vi "(SubVI) Guess Center xc yc From Raw FEC_YCC.vi"(5 "Enum":enum16{"parity method", "max-min method"}(ring), 6 "avg range for QPD center (nm)":dbl=600.0, 7 "QPD array (V)":dbl[](array[numeric]), 8 "Stage array(um)":dbl[](array[numeric]), 9 "Read data?":bool) -> (0 "Best Fit for min":cluster{"X":dbl[], "Best Polynomial Fit":dbl[]}, 1 "Best Fit for max":cluster{"X":dbl[], "Best Polynomial Fit":dbl[]}, 2 "Guess-QPD-center (V)":dbl, 3 "Guess-stage-center(um)":dbl)   [LabVIEW 2014]
uses:
  <vilib>/Analysis/6fits.llb/Curve Fitting Criteria.ctl
  <vilib>/Analysis/6fits.llb/General Linear Fit Algorithm.ctl
  <vilib>/Utility/file.llb/Read From Spreadsheet File (DBL).vi
  <vilib>/Analysis/NI_AALPro.lvlib
panel:
  out "Guess-stage-center by avg (um)":dbl
  out "Guess-stage-center by fit (um)":dbl
  out "Xm for min QPD":dbl
  out "Xm for max QPD":dbl
  in  "file path (dialog if empty)":path
  in  "Tab Control":T1(tab)
  out "Raw":cluster{"all rows":dbl[], "all rows":dbl[]}(graph)
  out "Fit":cluster{"all rows":dbl[], "all rows":dbl[]}(graph)
  out "Raw+Fit":cluster{"all rows":dbl[], "all rows":dbl[]}[](graph)
  out "XY Graph":T2(graph)
  out "Polynomial Coefficients":dbl[](array[numeric])
  out "Best Fit for QPD":dbl[](array[numeric])
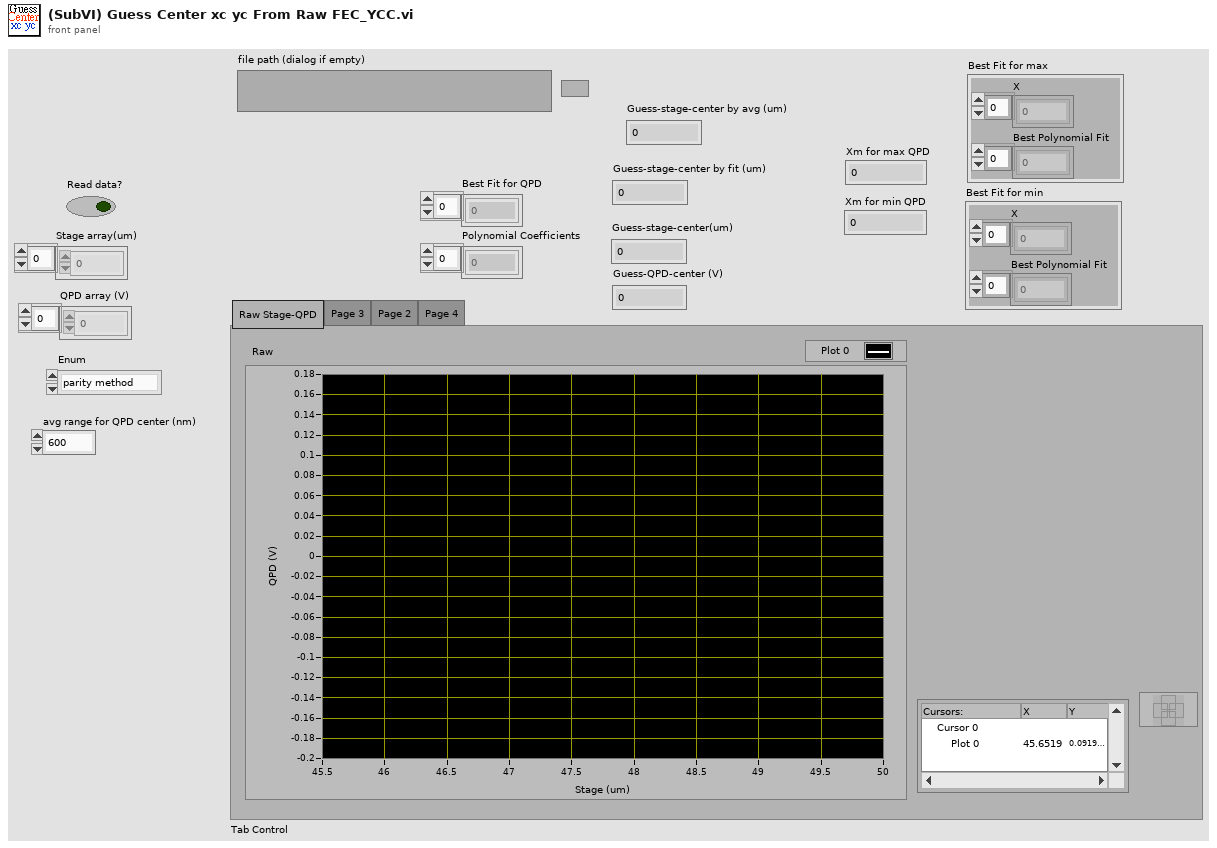
[diagram p1: front panel]
types:
  T1 = enum32{"Raw Stage-QPD", "Page 3", "Page 2", "Page 4"}
  T2 = cluster{"X":dbl[], "Best Polynomial Fit":dbl[]}[]
  T3 = typedef "NI_AALPro.lvlib/General Linear Fit Algorithm.ctl" = u16
  T4 = typedef "NI_AALPro.lvlib/Curve Fitting Criteria.ctl" = u16
  T5 = cluster{"all rows":dbl[], "Best Polynomial Fit":dbl[]}
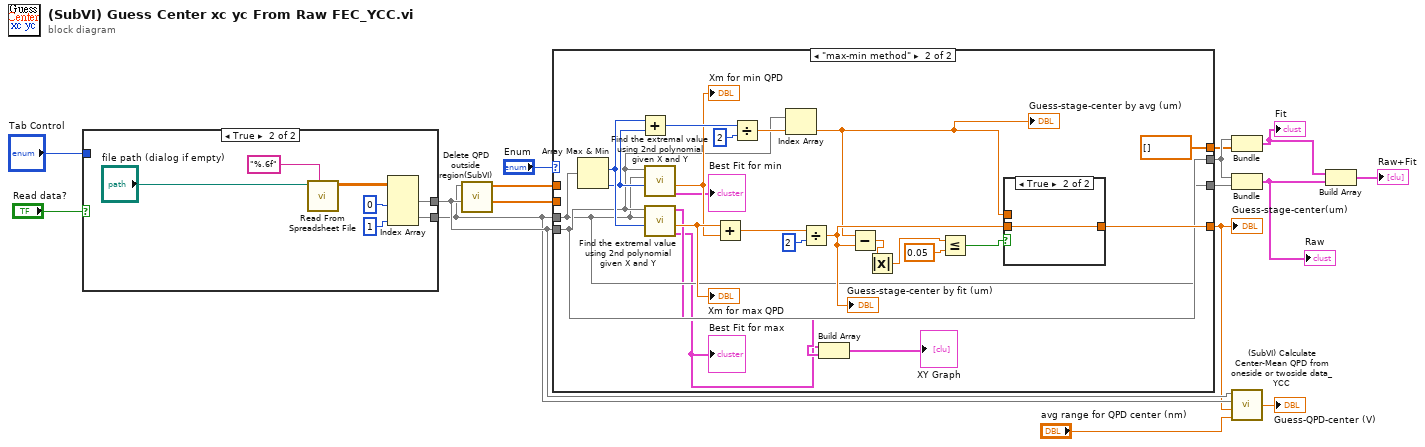
[diagram p0: block diagram]
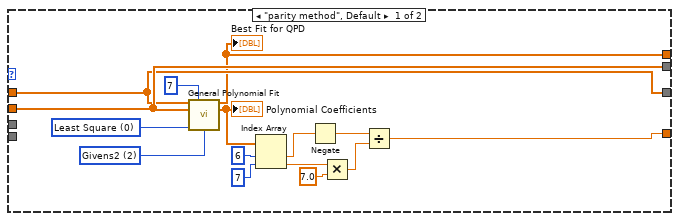
[diagram p2: hidden frame]
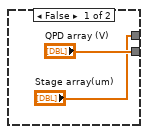
[diagram p4: hidden frame]
diagram:
  n1 = case shown="True" "Read data?" {
    tunnel: ["QPD array (V)" w20] -> w4
    tunnel: ["Stage array(um)" w21] -> w5
    tunnel: "Tab Control" -> [_ _]
    frame False {
    }
    frame True {
      n2 = call-poly <vilib>:"Read From Spreadsheet File.vi"("format (%.3f)"="%.6f", "file path (dialog if empty)"="file path (dialog if empty)") -> ("all rows"=w24:dbl[][])  [unwired: 5 in, 4 out]
      n3 = Index Array(array=w24, index (col) #1=0 ("disabled index (col)"), index (col) #2=1 ("index (col)")) -> (element #1=w21:dbl[], element #2=w20:dbl[])  [unwired: 2 in]
    }
  }
  n4 = call "Delete QPD outside region(SubVI).vi"("Position Array In"=w5, "QPD signal In"=w4) -> ("Position Array Out"=w14:dbl[], "QPD signal Out"=w13:dbl[])  [unwired: 8 in]
  n5 = case shown="\"max-min method\"" "Enum" {
    tunnel: w14 -> [w29 _]
    tunnel: w13 -> [w28 _]
    tunnel: w4 -> [_ w46]
    tunnel: w5 -> [_ w47]
    tunnel: [w26 w51] -> w3
    tunnel: [w29 w47] -> w9
    tunnel: [w28 w46] -> w10
    tunnel: [w27 dbl[] [] ("Best Polynomial Fit")] -> w8
    frame "parity method", Default {
      w30 = T3 2 items=["SVD", "Givens", "Givens2", "Householder", "LU Decomposition", "Cholesky", "SVD for Rank Deficient H"] ("algorithm")
      w31 = T4 0 items=["Least Square", "Least Absolute Residual", "Bisquare"] ("method")
      n6 = call <vilib>:"General Polynomial Fit.vi"("Y"=w28, "polynomial order"=7, "X"=w29, "method"=w31, "algorithm"=w30) -> ("Best Polynomial Fit"=w27:dbl[], "Polynomial Coefficients"=w39:dbl[])  [unwired: 7 in, 2 out]
      "Best Fit for QPD" <- w27
      "Polynomial Coefficients" <- w39
      n7 = Index Array(array=w39, index #1=6 ("index"), index #2=7 ("index")) -> (element #1=w36:dbl, element #2=w34:dbl)
      n8 = Negate(x=w36) -> (-x=w35:dbl)
      n9 = Multiply(x=w34, y=7.0) -> (x*y=w32:dbl)
      n10 = Divide(x=w35, y=w32) -> (x/y=w26:dbl)
    }
    frame "max-min method" {
      n11 = Array Max & Min(array=w46) -> (max index (indices)=w60:i32, min index (indices)=w59:i32)  [unwired: 2 out]
      n12 = Add(x=w60, y=w59) -> (x+y=w62:i32)
      n13 = call "Find the extremal value using 2nd polynomial given X and Y.vi"("initial guess index of X"=w59, "Y"=w46, "X"=w47) -> ("Best Fit"=→"Best Fit for min":cluster{"X":dbl[], "Best Polynomial Fit":dbl[]}, "Xm"=w55:dbl)  [unwired: 2 in, 1 out]
      "Xm for min QPD" <- w55
      n14 = call "Find the extremal value using 2nd polynomial given X and Y.vi"("initial guess index of X"=w60, "Y"=w46, "X"=w47) -> ("Best Fit"=w43:cluster{"X":dbl[], "Best Polynomial Fit":dbl[]}, "Xm"=w56:dbl, "input"=w44:cluster{"X":dbl[], "Best Polynomial Fit":dbl[]})  [unwired: 2 in]
      "Xm for max QPD" <- w56
      "Best Fit for max" <- w43
      n15 = Add(x=w56, y=w55) -> (x+y=w57:dbl)
      n16 = Divide(x=w62, y=2) -> (x/y=w61:dbl)
      n17 = Index Array(array=w47, index=w61) -> (element=w41:dbl)
      "Guess-stage-center by avg (um)" <- w41
      n18 = Divide(x=w57, y=2) -> (x/y=w50:dbl)
      "Guess-stage-center by fit (um)" <- w50
      n19 = Build Array(w43, w44) -> (→"XY Graph":T2)
      n20 = Subtract(x=w41, y=w50) -> (x-y=w49:dbl)
      n21 = Absolute Value(x=w49) -> (abs(x)=w48:dbl)
      n22 = Less Or Equal?(x=w48, y=0.05) -> (x <= y?=w52:bool)
      n23 = case shown="True" w52 {
        tunnel: w41 -> [w64 _]
        tunnel: w50 -> [_ w65]
        tunnel: [w64 w65] -> w51
        frame False {
        }
        frame True {
        }
      }
    }
  }
  "Guess-stage-center(um)" <- w3
  n24 = Bundle("all rows"=w9, "Best Polynomial Fit"=w8) -> (w6:T5)  [unwired: 1 in]
  "Fit" <- w6
  n25 = Bundle("all rows"=w9, "all rows"=w10) -> (w7:cluster{"all rows":dbl[], "all rows":dbl[]})  [unwired: 1 in]
  "Raw" <- w7
  n26 = call "(SubVI) Calculate Center-Mean QPD from oneside or twoside data_YCC.vi"("Stage Array (um)"=w5, "QPD Array (V)"=w4, "Center Stage (um)"=w3, "avg range for QPD center (nm)"="avg range for QPD center (nm)") -> ("Center QPD (V)"=→"Guess-QPD-center (V)":dbl)  [unwired: 3 in]
  n27 = Build Array(w6, w7) -> (→"Raw+Fit":cluster{"all rows":dbl[], "all rows":dbl[]}[])
